vi "Msg Send UI Message.vi"(5 "timeout in ms (-1)":i32=-1, 6 "error in (no error)":errorcluster, 7 "Data":variant, 8 "Message":string, 9 "user event":refnum<user-event>) -> (0 "error out":errorcluster, 1 "timed out?":bool, 2 "response":variant, 3 "user event":refnum<user-event>)   [LabVIEW 2014]
doc: "Send a message to the specified message queue (or event structure). This function awaits a response from the recipient which should be sent with Msg Send Response.vi.\n\nThis is part of the Msg suite, intended to make messaging architectures in LabVIEW\nSee the template \"Message Based Application Template.vi\" for normal usage.\n\nCopyright 2005-2016 Jason Sommerville\n\nSends a response to the original sender of a message (sent via Msg Send Message). It should form bookends with Msg Get Message in the message handling loop.\n\nThis is part of the Msg suite, intended to make messaging architectures in LabVIEW\nSee the template \"Message Based Application Template.vi\" for normal usage.\n\nCopyright 2005-2016 Jason Sommerville\n\nThis VI may be freely used, modified or distributed under the BSD license."
uses:
  Message Cluster.ctl
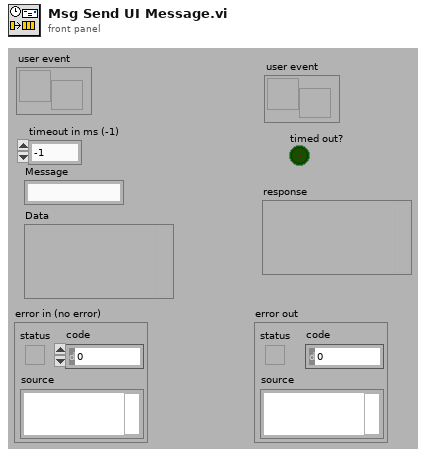
[diagram p1: front panel]
types:
  T1 = cluster{"Message":string, "Data":variant, "notifier out":refnum<notifier>}
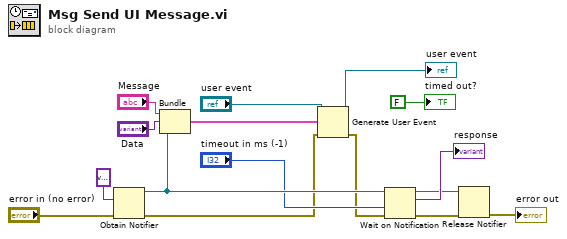
[diagram p0: block diagram]
diagram:
  n1 = Obtain Notifier(notification data type=variant ("Data"), error in (no error)="error in (no error)") -> (notifier out=w9:refnum<notifier>, error out=w3:errorcluster)  [unwired: 2 in, 1 out]
  n2 = Bundle("Message"="Message", "Data"="Data", "notifier out"=w9) -> (w12:T1)  [unwired: 1 in]
  n3 = Generate User Event(user event="user event", event data cluster=w12, error in=w3) -> (user event out=→"user event":refnum<user-event>, error out=w2:errorcluster)  [unwired: 1 in]
  n4 = Wait on Notification(notifier=w9, timeout in ms (-1)="timeout in ms (-1)", error in (no error)=w2) -> (notifier out=w5:refnum<notifier>, notification=→"response":variant, error out=w6:errorcluster)  [unwired: 1 in, 1 out]
  n5 = Release Notifier(notifier=w5, error in (no error)=w6) -> (error out=→"error out":errorcluster)  [unwired: 1 in, 2 out]
  "timed out?" <- FALSE ("timed out?")
